vi "Setup DMC TestRunner.vi"(4 "Exclude Bookmarks":string[](array[string]), 5 "Verbose":bool, 6 "Include Bookmarks":string[](array[string]), 7 "CLI":refnum<class "CLI.lvclass">, 8 "error in (no error)":errorcluster, 9 "Report Path":path, 10 "Paths":path[](array[path]), 11 "DMC Test Runner.Folder":refnum<class "DMC Folder Test Runner.lvclass">) -> (0 "error out":errorcluster, 3 "DMC Test Runner.Folder out":refnum<class "DMC Folder Test Runner.lvclass">)   [LabVIEW 2023, in "DMC Folder Test Runner.lvclass"]
uses:
  DMC Folder Test Runner.lvclass
  DMC Folder Test Runner.lvclass/DMC Folder Test Runner.ctl
  <vilib>/addons/_JKI Toolkits/Caraya/Caraya.lvlib
  <vilib>/addons/_JKI Toolkits/Caraya/classes/Test Runner.Folder/Test Runner.Folder.lvclass
  C:/Program Files/National Instruments/LabVIEW 2023/vi.lib/addons/_JKI Toolkits/Caraya/classes/Test Runner.Folder/Test Runner.Folder.lvclass
  C:/Program Files/National Instruments/LabVIEW 2023/vi.lib/addons/_JKI Toolkits/Caraya/classes/Test Runner/Test Runner.lvclass
  C:/projects/DMC/GitHub/DMC CLI Caraya/Source/DMC Folder Test Runner/DMC Folder Test Runner.lvclass
  <vilib>/Wiresmith Technology/G CLI/CLI Class/CLI.lvclass
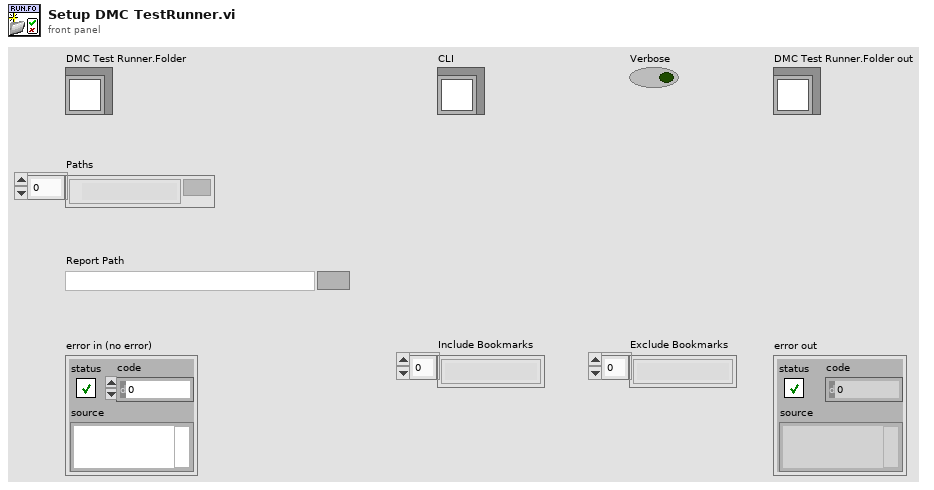
[diagram p1: front panel]
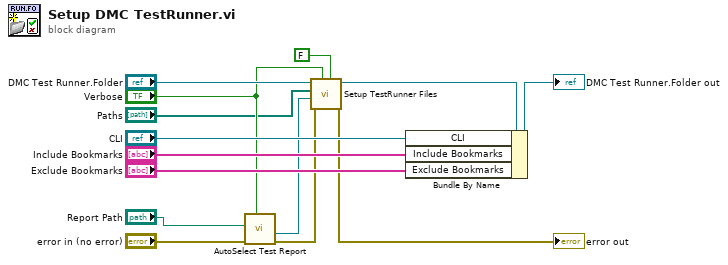
[diagram p0: block diagram]
diagram:
  n1 = call <vilib>:"AutoSelect Test Report.vi"("Verbose"="Verbose", "error in (no error)"="error in (no error)", "Report Path"="Report Path") -> ("error out"=w2:errorcluster, "Test Report out"=w3:refnum<class "Test Report.lvclass">)  [unwired: 7 in]
  n2 = call <vilib>:"Setup TestRunner Files.vi"("Interactive (T)"=FALSE, "Verbose (F)"="Verbose", "error in (no error)"=w2, "Test Report"=w3, "Paths"="Paths", "Test Runner.Folder"="DMC Test Runner.Folder") -> ("error out"=→"error out":errorcluster, "Test Runner.Folder out"=w7:refnum<class "DMC Folder Test Runner.lvclass">)  [unwired: 4 in]
  n3 = Bundle By Name(cluster=w7, "CLI"="CLI", "Include Bookmarks"="Include Bookmarks", "Exclude Bookmarks"="Exclude Bookmarks") -> (→"DMC Test Runner.Folder out":refnum<class "DMC Folder Test Runner.lvclass">)
